vi "Draw Intersection.vi"(8 "error in (no error)":errorcluster, 10 "Intersection Point":cluster{"X":sgl, "Y":sgl}, 11 "Refnum in":T1) -> (0 "error out":errorcluster, 3 "Refnum out":T1)   [LabVIEW 2017]
uses:
  <vilib>/vision/Image Controls.llb/IMAQ Image.ctl
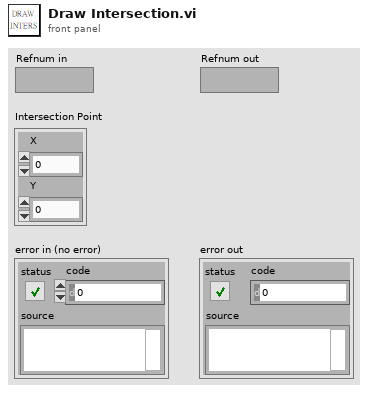
[diagram p1: front panel]
types:
  T1 = typedef "IMAQ Image.ctl" = refnum<image>
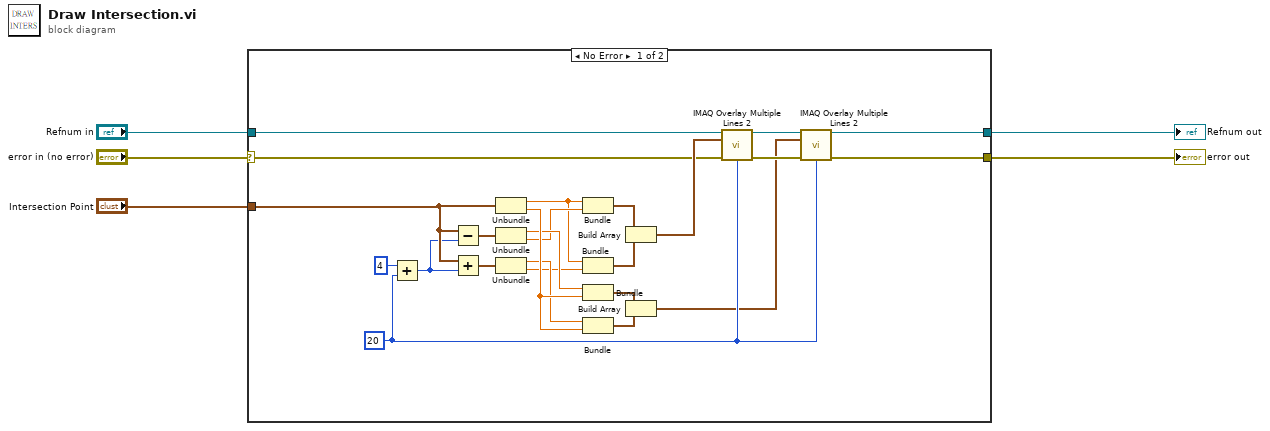
[diagram p0: block diagram]
diagram:
  n1 = case shown="No Error" "error in (no error)" {
    selector: "error in (no error)" -> [w6 w31]
    tunnel: [w29 w31] -> w5
    tunnel: [w26 w30] -> w4
    tunnel: "Refnum in" -> [w25 w30]
    tunnel: "Intersection Point" -> [w24 _]
    frame No Error {
      w27 = u32 20 ("Width")
      n2 = Add(x=u32 4, y=w27) -> (x+y=w22:u32)
      n3 = Subtract(x=w24, y=w22) -> (x-y=w8:cluster{"X":sgl, "Y":sgl})
      n4 = Add(x=w24, y=w22) -> (x+y=w9:cluster{"X":sgl, "Y":sgl})
      n5 = Unbundle(w24) -> ("X"=w10:sgl, "Y"=w18:sgl)
      n6 = Unbundle(w8) -> ("X"=w16:sgl, "Y"=w11:sgl)
      n7 = Unbundle(w9) -> ("X"=w17:sgl, "Y"=w12:sgl)
      n8 = Bundle("X"=w10, "Y"=w11) -> (w13:cluster{"X":sgl, "Y":sgl})  [unwired: 1 in]
      n9 = Bundle("X"=w10, "Y"=w12) -> (w14:cluster{"X":sgl, "Y":sgl})  [unwired: 1 in]
      n10 = Bundle("X"=w16, "Y"=w18) -> (w19:cluster{"X":sgl, "Y":sgl})  [unwired: 1 in]
      n11 = Bundle("X"=w17, "Y"=w18) -> (w20:cluster{"X":sgl, "Y":sgl})  [unwired: 1 in]
      n12 = Build Array(w13, w14) -> (w15:cluster{"X":sgl, "Y":sgl}[])
      n13 = Build Array(w19, w20) -> (w21:cluster{"X":sgl, "Y":sgl}[])
      n14 = call "IMAQ Overlay Multiple Lines 2"("Image"=w25, "Line End Points"=w15, "error in (no error)"=w6, "Width"=w27) -> ("Image Out"=w7:T1, "error out"=w28:errorcluster)  [unwired: 10 in]
      n15 = call "IMAQ Overlay Multiple Lines 2"("Image"=w7, "Line End Points"=w21, "error in (no error)"=w28, "Width"=w27) -> ("Image Out"=w26:T1, "error out"=w29:errorcluster)  [unwired: 10 in]
    }
    frame Error {
    }
  }
  "error out" <- w5
  "Refnum out" <- w4
